vi "GOOP_MyComputer_CreateNewWizard_Invoke.vi"(10 "New Item Parent":T1, 11 "Wizard":u64) -> (3 "Canceled":bool)   [LabVIEW 2020]
uses:
  <resource>/Framework/Providers/API/mxLvNIIM.ctl
  <resource>/Framework/Providers/Open_GDS/SubVIs/GOOP_ClassProviderClassType.ctl
  <resource>/Framework/Providers/Open_GDS/ClassProviders/Provider_BaseClassInterface/ClassWriter_class/ClassWriter.lvclass
  <resource>/Framework/Providers/Open_GDS/ClassProviders/Common/InterfaceLibrary/InterfaceLibrary.lvlib
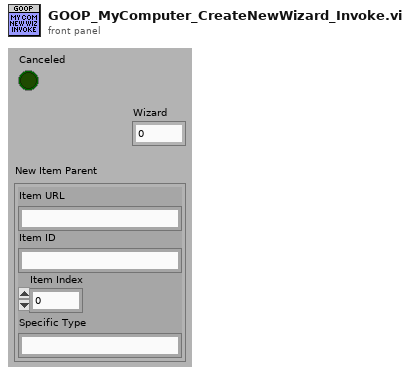
[diagram p1: front panel]
types:
  T1 = typedef "mxLvNIIM.ctl" = cluster{"Item URL":string, "Item ID":string, "Item Index":i32, "Specific Type":string}
  T2 = typedef "GOOP_ClassProviderClassType.ctl" = enum16{"ClassWriter", "ClassReader"}
  T3 = typedef "ClassWriter.lvclass/InterfacesToImplement.ctl" = cluster{"InterfacePath":path[], "CreateMethods":bool, "MethodsPerInterface(Empty=>All)":cluster{"Methods":string[]}[]}
  T4 = typedef "ClassWriter.lvclass/CreateClassData.ctl" = cluster{"ClassName":string, "ClassFolder":path, "ClassDescription":string, "ClassTemplateOptions":string, "BaseClass(ProjectStringPath or LvClassFilePath)":variant, "ExtraCreateParameters":variant, "FolderSuffix":string, "ParentInterfaces":path[]}
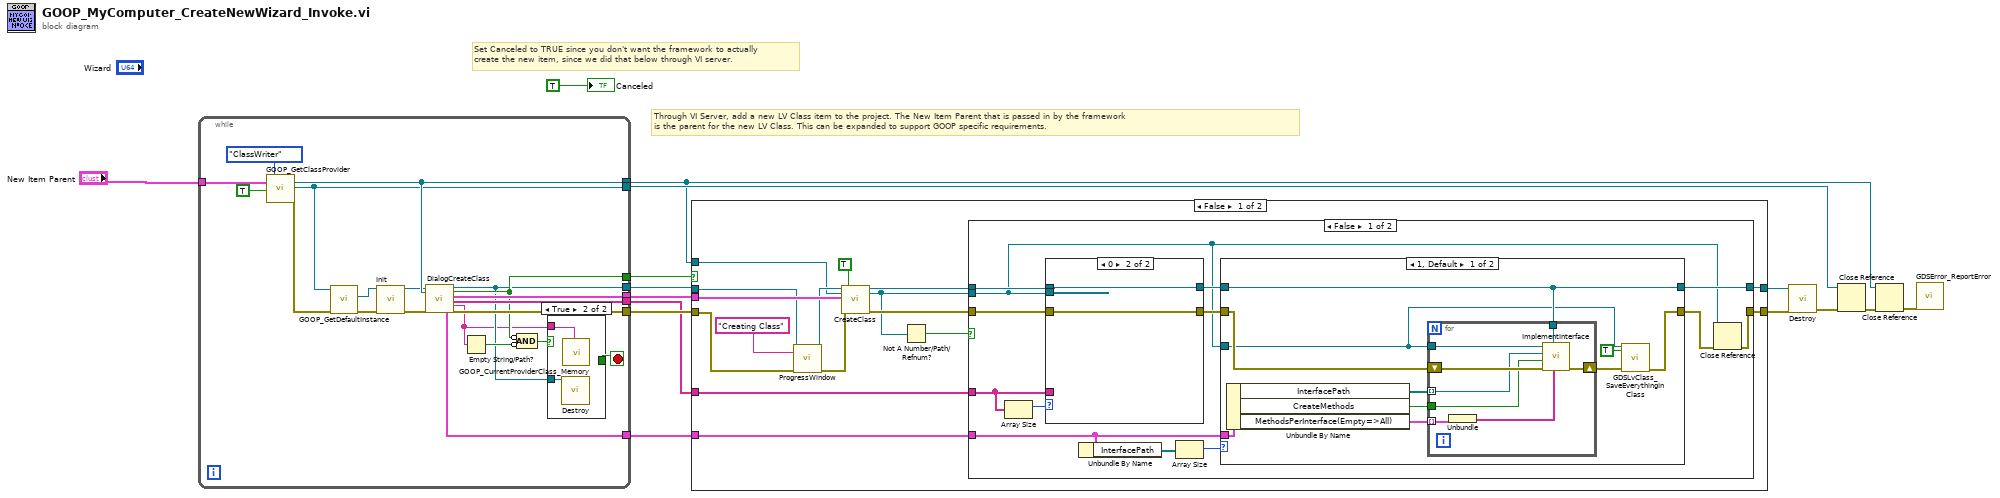
[diagram p0: block diagram]
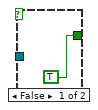
[diagram p2: hidden frame]
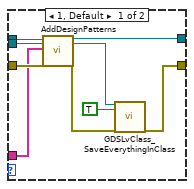
[diagram p4: hidden frame]
diagram:
  # "Through VI Server, add a new LV Class item to the project. The New Item Parent that is passed in by the framework\nis the parent for the new LV Class. This can be expanded to support GOOP specific requirements."
  # "Set Canceled to TRUE since you don't want the framework to actually\ncreate the new item, since we did that below through VI server."
  n1 = while {
    tunnel: "New Item Parent" -> [w35]
    tunnel: [w18] -> w8
    tunnel: [w34] -> w10
    tunnel: [w33] -> w9
    tunnel: [w31] -> w7
    tunnel: [w26] -> w11
    tunnel: [w23] -> w6
    tunnel: [w22] -> w2
    tunnel: [w16] -> w1
    stop <- w19 stop-if-true
    n2 = call <resource>:"GOOP_GetClassProvider.vi"("New Item Parent/Object"=w35, "CreateClass"=TRUE, "ProviderClassType"=GOOP_ClassProviderClassType."ClassWriter") -> ("ProjectItem"=w31:refnum<vi>, "LVClass.Open"=w26:refnum<vi>, "error out"=w25:errorcluster)  [unwired: 14 in]
    n3 = call <resource>:"GOOP_GetDefaultInstance.vi"("error in"=w25, "LVClassIn"=w26) -> ("error out"=w27:errorcluster, "ClassWriter.lvclass"=w24:refnum<class "ClassWriter.lvclass">)  [unwired: 7 in, 1 out]
    n4 = call-dynamic "Init.vi"("ClassWriter in"=w24, "error in (no error)"=w27) -> ("ClassWriter out"=w29:refnum<class "ClassWriter.lvclass">, "error out"=w28:errorcluster)  [unwired: 16 in]
    n5 = call-dynamic "DialogCreateClass.vi"("ClassWriter in"=w29, "ProjectItem Refnum"=w31, "error in (no error)"=w28) -> ("InterfaceToImplement"=w16:T3, "ClassWriter out"=w18:refnum<class "ClassWriter.lvclass">, "Cancelled"=w22:bool, "CreateClassData"=w33:T4, "DesignPatternsToAddAfterCreation"=w23:string[], "ChangeProviderRequested"=w17:string, "error out"=w34:errorcluster)  [unwired: 10 in]
    n6 = Empty String/Path?(string/path=w17) -> (empty?=w21:bool)
    n7 = Compound Arithmetic op=AND(invert w22, invert w21) -> (w20:bool)
    n8 = case shown="True" w20 {
      tunnel: w17 -> [_ w38]
      tunnel: [TRUE _] -> w19
      tunnel: w18 -> [_ w37]
      frame False {
      }
      frame True {
        n9 = call-dynamic "Destroy.vi"("ClassWriter.lvclass"=w37) -> ()  [unwired: 18 in, 1 out]
        n10 = call <resource>:"GOOP_CurrentProviderClass_Memory.vi"("SetDefaultClassProvider(Ignored if not wired)"=w38) -> ()  [unwired: 12 in, 7 out]
      }
    }
  }
  n11 = case shown="False" w2 {
    tunnel: w8 -> [w53 w101]
    tunnel: w10 -> [w39 w102]
    tunnel: w7 -> [w46 _]
    tunnel: [w44 w102] -> w4
    tunnel: w9 -> [w54 _]
    tunnel: [w48 w101] -> w5
    tunnel: w6 -> [w47 _]
    tunnel: w1 -> [w41 _]
    frame False {
      n12 = call-dynamic "ProgressWindow.vi"("ClassWriter in"=w53, "Message(Exit)"="Creating Class", "error in (no error)"=w39) -> ("ClassWriter out"=w52:refnum<class "ClassWriter.lvclass">, "error out"=w51:errorcluster)  [unwired: 15 in]
      n13 = call-dynamic "CreateClass.vi"("ClassWriter.lvclass"=w52, "ProjectTreePosition(String or Project Item Ref)"=w46, "CreateClassData"=w54, "error in (no error)"=w51, "KeepLvClassRefOpen(False)"=TRUE) -> ("ClassWriter.lvclass"=w50:refnum<class "ClassWriter.lvclass">, "LVClassLibraryRefnum"=w43:refnum<vi>, "error out"=w49:errorcluster)  [unwired: 11 in, 1 out]
      n14 = Not A Number/Path/Refnum?(number/path/refnum=w43) -> (NaN/Path/Refnum?=w42:bool)
      n15 = case shown="False" w42 {
        tunnel: w50 -> [w66 w100]
        tunnel: w49 -> [w65 w99]
        tunnel: [w59 w100] -> w48
        tunnel: w47 -> [w64 _]
        tunnel: [w63 w99] -> w44
        tunnel: w43 -> [w56 _]
        tunnel: w41 -> [w55 _]
        frame False {
          n16 = Array Size(array=w64) -> (size(s)=w67:i32)
          n17 = case shown="0" w67 {
            tunnel: w66 -> [w96 w98]
            tunnel: w65 -> [w95 w97]
            tunnel: [w88 w97] -> w58
            tunnel: [w94 w98] -> w60
            tunnel: w64 -> [w93 _]
            tunnel: w56 -> [w92 _]
            frame 1, Default {
              n18 = call-dynamic "AddDesignPatterns.vi"("ClassWriterNative"=w96, "ClassItemRefIn"=w92, "DesignPatterns"=w93, "error in (no error)"=w95) -> ("ClassWriterNative"=w94:refnum<class "ClassWriter.lvclass">, "ClassItemRefOut"=w90:refnum<vi>, "error out"=w89:errorcluster)  [unwired: 12 in, 1 out]
              n19 = call <resource>:"GDSLvClass_SaveEverythingInClass.vi"("ClassRefIn"=w90, "ForceResaving(False)"=TRUE, "error in"=w89) -> ("error out"=w88:errorcluster)  [unwired: 15 in, 1 out]
            }
            frame 0 {
            }
          }
          n20 = Unbundle By Name(w55) -> ("InterfacePath"=w62:path[])
          n21 = Array Size(array=w62) -> (size(s)=w61:i32)
          n22 = case shown="1, Default" w61 {
            tunnel: w60 -> [w69 w87]
            tunnel: w58 -> [w75 w86]
            tunnel: [w76 w86] -> w57
            tunnel: [w69 w87] -> w59
            tunnel: w56 -> [w68 _]
            tunnel: w55 -> [w74 _]
            frame 1, Default {
              n23 = Unbundle By Name(w74) -> ("InterfacePath"=w73:path[], "CreateMethods"=w72:bool, "MethodsPerInterface(Empty=>All)"=w71:cluster{"Methods":string[]}[])
              n24 = for {
                tunnel: w68 -> [w85]
                tunnel: w73 -> [w83] mode=indexing
                tunnel: w72 -> [w82]
                tunnel: w71 -> [w81] mode=indexing
                shift-right: [w79] -> w70
                shift-left: w75 -> [w84]
                tunnel: w69 -> [w78]
                n25 = Unbundle(w81) -> ("Methods"=w80:string[])
                n26 = call <resource>:"ImplementInterface.vi"("InterfaceMethodsToCreate"=w80, "ClassWriter.lvclass"=w78, "error in"=w84, "CreateMethods"=w82, "Interface Path"=w83, "LvClassPath/LvClassProjectItem"=w85) -> ("error out"=w79:errorcluster)  [unwired: 5 in]
              }
              n27 = call <resource>:"GDSLvClass_SaveEverythingInClass.vi"("ClassRefIn"=w68, "ForceResaving(False)"=TRUE, "error in"=w70) -> ("error out"=w76:errorcluster)  [unwired: 15 in, 1 out]
            }
            frame 0 {
            }
          }
          n28 = Close Reference(reference=w56, error in (no error)=w57) -> (error out=w63:errorcluster)
        }
        frame True {
        }
      }
    }
    frame True {
    }
  }
  n29 = call-dynamic "Destroy.vi"("ClassWriter.lvclass"=w5, "error in (no error)"=w4) -> ("error out"=w14:errorcluster)  [unwired: 17 in]
  n30 = Close Reference(reference=w11, error in (no error)=w14) -> (error out=w13:errorcluster)
  n31 = Close Reference(reference=w7, error in (no error)=w13) -> (error out=w12:errorcluster)
  n32 = call <resource>:"GDSError_ReportError.vi"("error in (no error)"=w12) -> ()  [unwired: 18 in, 1 out]
  "Canceled" <- TRUE ("Canceled")
